vi "Teleop Shooter Control.vi"(8 "Manipulator D-Pad":T1, 9 "Manipulator Buttons":T2, 10 "Driver Buttons":T2) -> ()   [LabVIEW 2015]
uses:
  Common Code/Gamepads/Button Cluster.ctl
  Common Code/Gamepads/D-Pad.ctl
  Common Code/Shooter Commands.ctl
  Common Code/Shot Type.ctl
  Robot Global Data.vi
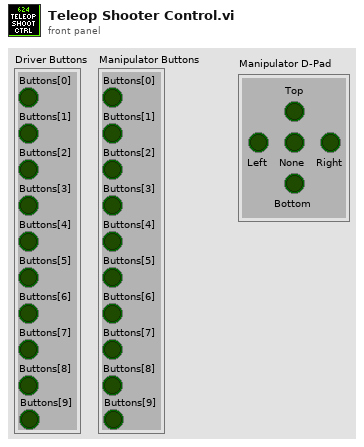
[diagram p1: front panel]
types:
  T1 = typedef "D-Pad.ctl" = cluster{"Top":bool, "Bottom":bool, "None":bool, "Right":bool, "Left":bool}
  T2 = typedef "Button Cluster.ctl" = cluster{"Buttons[0]":bool, "Buttons[1]":bool, "Buttons[2]":bool, "Buttons[3]":bool, "Buttons[4]":bool, "Buttons[5]":bool, "Buttons[6]":bool, "Buttons[7]":bool, "Buttons[8]":bool, "Buttons[9]":bool}
  T3 = typedef "Shooter Command Cluster.ctl" = cluster{"Command":T4, "Mode":T5, "Shot Type":T6}
  T4 = typedef "Shooter Commands.ctl" = enum16{"Idle", "Prime Shooter", "Shoot"}
  T5 = typedef "Shoot Modes Enum.ctl" = enum16{"Manual", "Safe", "Auto"}
  T6 = typedef "Shot Type.ctl" = enum16{"Batter Shot", "Curve Shot", "Vision Shot", "Deep Middle Shot"}
  T7 = typedef "Manual Shoot.ctl" = cluster{"Spin Wheels":bool, "Fire":bool}
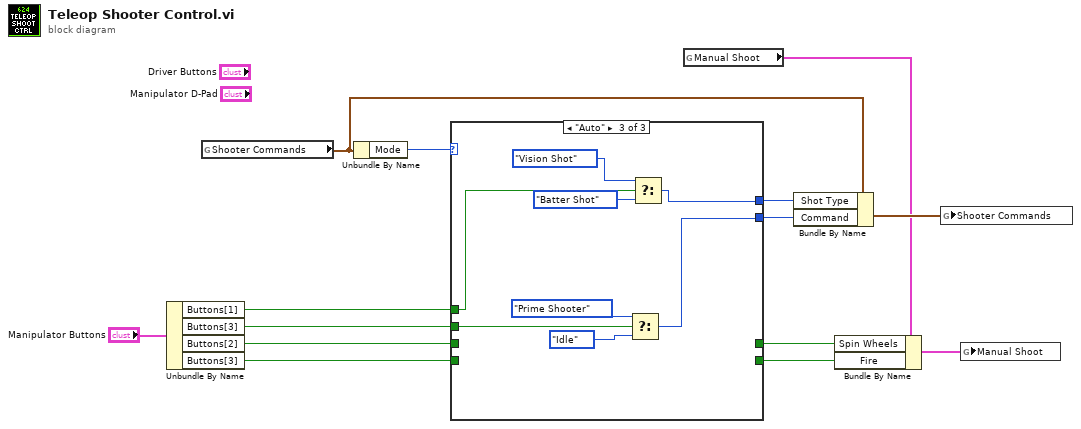
[diagram p0: block diagram]
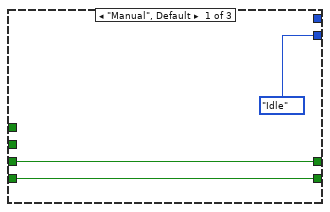
[diagram p2: hidden frame]
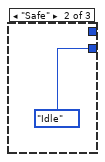
[diagram p3: hidden frame]
diagram:
  n1 = Unbundle By Name("Manipulator Buttons") -> ("Buttons[1]"=w11:bool, "Buttons[3]"=w12:bool, "Buttons[2]"=w7:bool, "Buttons[3]"=w1:bool)
  n2 = global read "Robot Global Data.vi" "Shooter Commands"() -> (w9:T3)
  n3 = Unbundle By Name(w9) -> ("Mode"=w8:T5)
  n4 = case shown="\"Auto\"" w8 {
    tunnel: w12 -> [_ _ w26]
    tunnel: w11 -> [_ _ w22]
    tunnel: [Shooter_Commands."Idle" ("Command") Shooter_Commands."Idle" ("Command") w23] -> w10
    tunnel: w7 -> [w16 _ _]
    tunnel: [w16 _ _] -> w5
    tunnel: [w15 _ _] -> w3
    tunnel: w1 -> [w15 _ _]
    tunnel: [_ _ w20] -> w2
    frame "Manual", Default {
    }
    frame "Safe" {
    }
    frame "Auto" {
      n5 = Select(t=Shooter_Commands."Prime Shooter" ("Command"), s=w26, f=Shooter_Commands."Idle" ("Command")) -> (s? t:f=w23:T4)
      n6 = Select(t=Shot_Type."Vision Shot" ("Shot Type"), s=w22, f=Shot_Type."Batter Shot") -> (s? t:f=w20:T6)
    }
  }
  n7 = global read "Robot Global Data.vi" "Manual Shoot"() -> (w6:T7)
  n8 = Bundle By Name(cluster=w9, "Shot Type"=w2, "Command"=w10) -> (w13:T3)
  n9 = Bundle By Name(cluster=w6, "Spin Wheels"=w5, "Fire"=w3) -> (w4:T7)
  n10 = global write "Robot Global Data.vi" "Shooter Commands"(w13) -> ()
  n11 = global write "Robot Global Data.vi" "Manual Shoot"(w4) -> ()
